vi "Create Test Configuration.vi"() -> (0 "error out":errorcluster, 1 "Channel Names":string[](array[string]), 2 "Array":refnum<class "TBM channel.lvclass">[](array[class]), 3 "TEC configuration out":refnum<class "TEC configuration.lvclass">)   [LabVIEW 2014, in "TEC tests.lvlib"]
uses:
  TEC tests.lvlib
  <vilib>/NI/Tag Bus Module Framework/channel/TBM channel.lvclass
  configuration/TEC configuration.lvclass
  <vilib>/NI/Tag Bus Module Framework/channel/channel classification.ctl
  configuration/TEC configuration.lvclass/TEC configuration.ctl
  configuration/Write channels.vi
  <vilib>/NI/Configuration Framework/serializable configuration/NISE_CEF_serializable configuration.lvclass
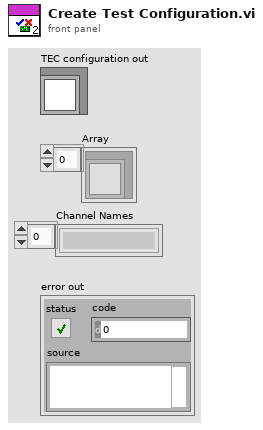
[diagram p1: front panel]
types:
  T1 = typedef "TBM channel.lvclass/channel classification.ctl" = enum16{"input data", "output data", "processing parameter", "processing result"}
  T2 = typedef "tag bus.lvlib/tag descriptor.lvclass/Data Type.ctl" = enum16{"Double", "Single", "I64", "I32", "I16", "I8", "U64", "U32", "U16", "U8", "Boolean", "String", "Array of Double", "Array of Single", "Array of I64", "Array of I32", "Array of I16", "Array of I8", "Array of U64", "Array of U32", "Array of U16", "Array of U8", "Array of Boolean", "Array of String"}
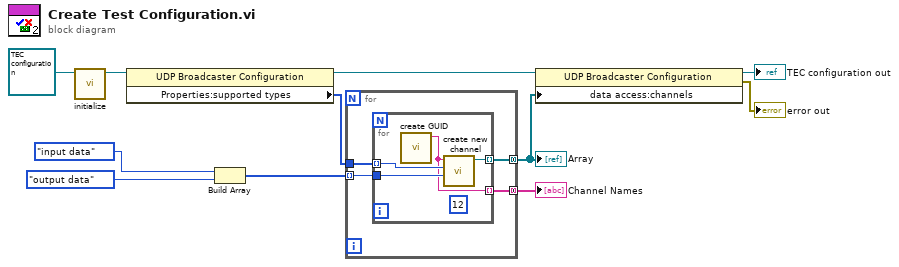
[diagram p0: block diagram]
diagram:
  n1 = call <vilib>:"initialize.vi"("configuration in"=refnum<class "TEC configuration.lvclass"> refnum ("tag bus configurable plugin module configuration")) -> ("configuration out"=w2:refnum<class "TEC configuration.lvclass">)  [unwired: 8 in, 2 out]
  n2 = property class="UDP Broadcaster Configuration"(reference=w2) -> (reference out=w8:refnum<class "TEC configuration.lvclass">, "Properties:supported types"=w7:T2[])  [unwired: 1 in, 1 out]
  n3 = Build Array(channel_classification."input data" ("channel classification"), channel_classification."output data" ("channel classification")) -> (w6:T1[])
  n4 = for {
    tunnel: w6 -> [w15] mode=indexing
    tunnel: [w14] -> w10 mode=concatenating
    tunnel: w7 -> [w13]
    tunnel: [w12] -> w1 mode=concatenating
    n5 = for {
      tunnel: w15 -> [w18]
      tunnel: [w19] -> w14 mode=indexing
      tunnel: w13 -> [w17] mode=indexing
      tunnel: [w16] -> w12 mode=indexing
      (unwired) 12
      n6 = call <vilib>:"create GUID.vi"() -> ("uuid"=w16:string)  [unwired: 10 in, 1 out]
      n7 = call <vilib>:"create new channel.vi"("channel classification"=w18, "data type"=w17, "channel name"=w16) -> ("channel"=w19:refnum<class "TBM channel.lvclass">)  [unwired: 8 in]
    }
  }
  "Array" <- w10
  "Channel Names" <- w1
  n8 = property class="UDP Broadcaster Configuration"(reference=w8, "data access:channels"=w10) -> (reference out=→"TEC configuration out":refnum<class "TEC configuration.lvclass">, error out=→"error out":errorcluster)  [unwired: 1 in]
